vi "test.StringHistoryCacher.vi"() -> ()   [LabVIEW 2017]
panel:
  out "String":string
  in  "stop":bool
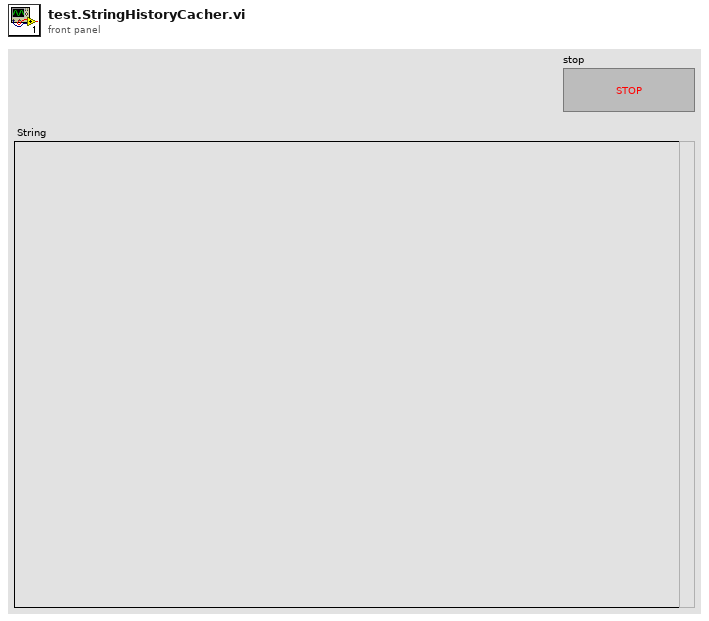
[diagram p1: front panel]
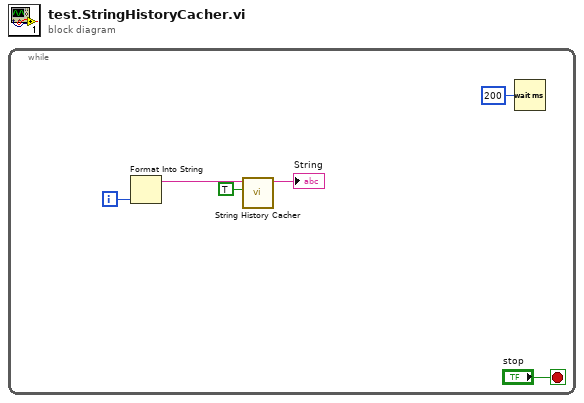
[diagram p0: block diagram]
diagram:
  n1 = while {
    i -> [w4]
    stop <- "stop" stop-if-true
    n2 = Format Into String(w4) -> (resulting string=w3:string)  [unwired: 3 in, 1 out]
    n3 = call "String History Cacher.vi"("Include Timestamp(F)"=TRUE, "String"=w3) -> ("String Cache"=→"String":string)  [unwired: 9 in]
    n4 = Wait (ms)(milliseconds to wait=u32 200) -> ()  [unwired: 1 out]
  }
